vi "Tank Drive.vi"   [LabVIEW 2013]
types:
  T1 = typedef "Right Drive Joystick.ctl" = cluster{"Buttons":T2, "Axes":cluster{"axis 1 (x)":dbl, "axis 2 (y)":dbl, "axis 3 (throttle)":dbl, "axis 4":dbl, "axis 5":dbl, "axis 6":dbl}}
  T2 = typedef "WPI_JoystickButtonState.ctl" = cluster{"Button 1":bool, "Button 2":bool, "Button 3":bool, "Button 4":bool, "Button 5":bool, "Button 6":bool, "Button 7":bool, "Button 8":bool, "Button 9":bool, "Button 10":bool, "Button 11":bool, "Button 12":bool}
  T3 = typedef "Left Drive Joystick.ctl" = cluster{"Buttons":T2, "Axes":cluster{"axis 1 (x)":dbl, "axis 2 (y)":dbl, "axis 3 (throttle)":dbl, "axis 4":dbl, "axis 5":dbl, "axis 6":dbl}}
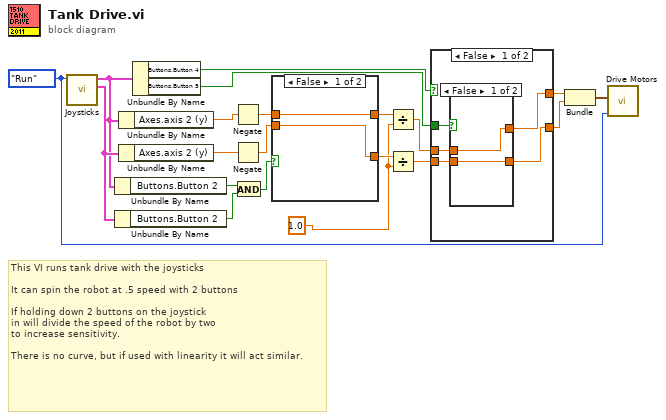
[diagram p0: block diagram]
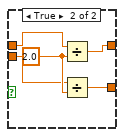
[diagram p2: hidden frame]
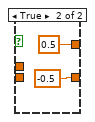
[diagram p3: hidden frame]
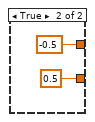
[diagram p4: hidden frame]
diagram:
  w1 = 1.0 ("y")
  w7 = enum16{"Init", "Run", "End"}."Run" ("Mode")
  # "This VI runs tank drive with the joysticks\n\nIt can spin the robot at .5 speed with 2 buttons\n\nIf holding down 2 buttons on the joystick\nin will divide the speed of the robot by two\nto increase sensitivity.\n\nThere is no curve, but if used with linearity it will act similar."
  n1 = call "Joysticks.vi"("Mode"=w7) -> ("Right Driving Joystick Values"=w18:T1, "Left Driving Joystick Values"=w17:T3)  [unwired: 7 out]
  n2 = Unbundle By Name(w17) -> ("Buttons.Button 2"=w16:bool)
  n3 = Unbundle By Name(w18) -> ("Buttons.Button 2"=w15:bool)
  n4 = Unbundle By Name(w17) -> ("Axes.axis 2 (y)"=w13:dbl)
  n5 = Unbundle By Name(w18) -> ("Axes.axis 2 (y)"=w12:dbl)
  n6 = Unbundle By Name(w17) -> ("Buttons.Button 4"=w19:bool, "Buttons.Button 5"=w20:bool)
  n7 = Negate(x=w13) -> (-x=w3:dbl)
  n8 = Negate(x=w12) -> (-x=w2:dbl)
  n9 = And(x=w16, y=w15) -> (x .and. y?=w14:bool)
  n10 = case shown="False" w14 {
    tunnel: w3 -> [w22 w26]
    tunnel: w2 -> [w21 w25]
    tunnel: [w22 w24] -> w11
    tunnel: [w21 w23] -> w10
    frame False {
    }
    frame True {
      w27 = 2.0 ("y")
      n11 = Divide(x=w26, y=w27) -> (x/y=w24:dbl)
      n12 = Divide(x=w25, y=w27) -> (x/y=w23:dbl)
    }
  }
  n13 = Divide(x=w11, y=w1) -> (x/y=w9:dbl)
  n14 = Divide(x=w10, y=w1) -> (x/y=w8:dbl)
  n15 = case shown="False" w19 {
    tunnel: w20 -> [w32 _]
    tunnel: w9 -> [w31 _]
    tunnel: w8 -> [w30 _]
    tunnel: [w29 0.5 ("Right In")] -> w4
    tunnel: [w28 -0.5 ("Left In")] -> w5
    frame False {
      n16 = case shown="False" w32 {
        tunnel: w31 -> [w33 _]
        tunnel: w30 -> [w34 _]
        tunnel: [w34 -0.5 ("Right In")] -> w29
        tunnel: [w33 0.5 ("Left In")] -> w28
        frame False {
        }
        frame True {
        }
      }
    }
    frame True {
    }
  }
  n17 = Bundle("Left In"=w5, "Right In"=w4) -> (w6:cluster{"Left In":dbl, "Right In":dbl})  [unwired: 1 out]
  n18 = call "Drive Motors.vi"("Mode"=w7, "Inputs"=w6) -> ()  [unwired: 2 in, 8 out]
